vi "Condition.vi"(8 "error in (no error)":errorcluster, 11 "Measurement3D in":refnum<class "Measurement3D.lvclass">) -> (0 "error out":errorcluster, 2 "Finish?":bool, 3 "Measurement3D out":refnum<class "Measurement3D.lvclass">)   [LabVIEW 2014, in "Measurement3D.lvclass"]
uses:
  Measurement3D.lvclass
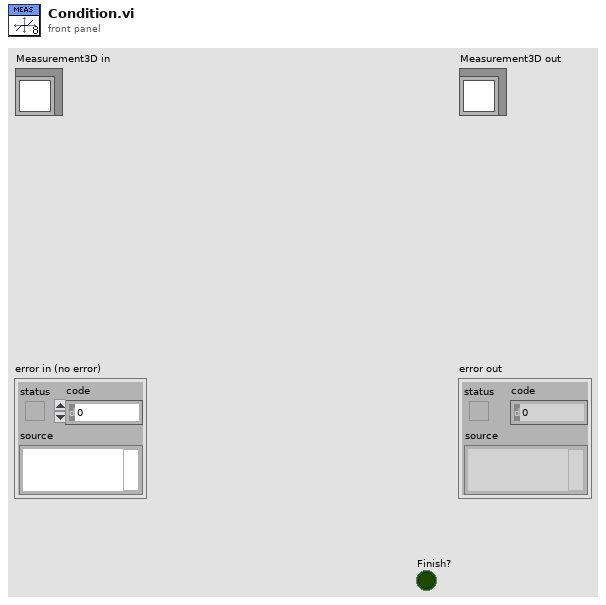
[diagram p1: front panel]
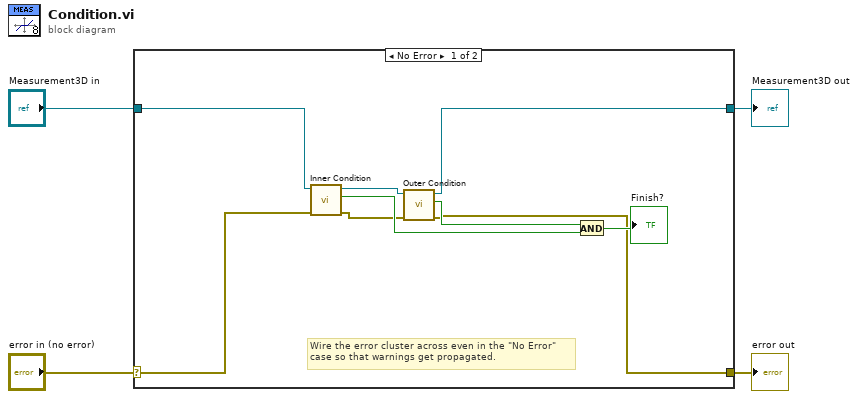
[diagram p0: block diagram]
diagram:
  n1 = case shown="No Error" "error in (no error)" {
    selector: "error in (no error)" -> [w8 w15]
    tunnel: [w6 w15] -> w3
    tunnel: [w5 w14] -> w1
    tunnel: "Measurement3D in" -> [w12 w14]
    frame No Error {
      # "Wire the error cluster across even in the \"No Error\"\ncase so that warnings get propagated."
      n2 = call "Inner Condition.vi"("error in (no error)"=w8, "Measurement3D in"=w12) -> ("error out"=w7:errorcluster, "Finish?"=w9:bool, "Measurement3D out"=w11:refnum<class "Measurement3D.lvclass">)  [unwired: 7 in]
      n3 = call "Outer Condition.vi"("error in (no error)"=w7, "Measurement3D in"=w11) -> ("error out"=w6:errorcluster, "Finish?"=w10:bool, "Measurement3D out"=w5:refnum<class "Measurement3D.lvclass">)  [unwired: 7 in]
      n4 = And(x=w10, y=w9) -> (x .and. y?=→"Finish?":bool)
    }
    frame Error {
    }
  }
  "error out" <- w3
  "Measurement3D out" <- w1
